vi "Get Wfm Logs.vi"(8 "error in (no error)":errorcluster, 11 "Waveform Receive in":refnum<class "Waveform Receive.lvclass">) -> (0 "error out":errorcluster, 2 "Associated Logs":T1[](array[typedef]), 3 "Waveform Receive out":refnum<class "Waveform Receive.lvclass">)   [LabVIEW 2015, in "Waveform Receive.lvclass"]
uses:
  Waveform Receive.lvclass
  Associated Log.ctl
  Waveform Receive.lvclass/Waveform Receive.ctl
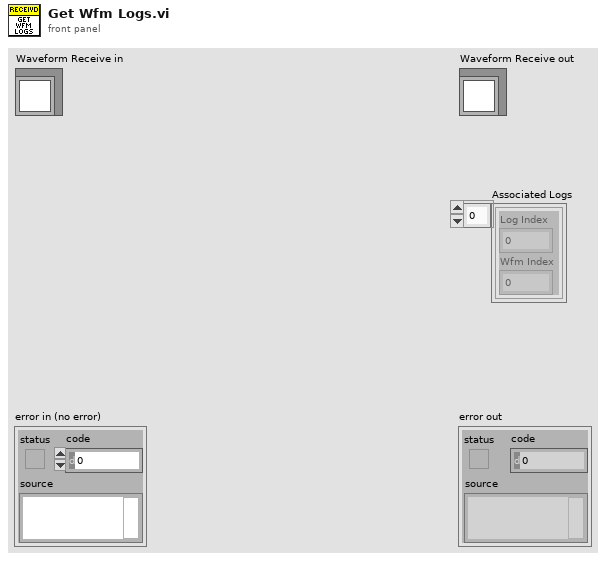
[diagram p1: front panel]
types:
  T1 = typedef "Waveform Receive.lvclass/Associated Log.ctl" = cluster{"Log Index":i32, "Wfm Index":i32}
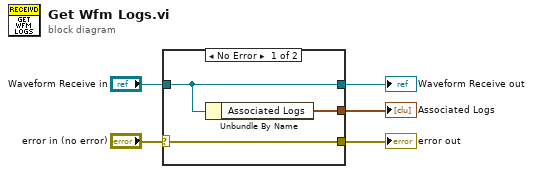
[diagram p0: block diagram]
diagram:
  n1 = case shown="No Error" "error in (no error)" {
    selector: "error in (no error)" -> [w8 w10]
    tunnel: [w8 w10] -> w4
    tunnel: [w7 w9] -> w2
    tunnel: "Waveform Receive in" -> [w7 w9]
    tunnel: [w6 _] -> w1
    frame No Error {
      n2 = Unbundle By Name(w7) -> ("Associated Logs"=w6:T1[])
    }
    frame Error {
    }
  }
  "error out" <- w4
  "Waveform Receive out" <- w2
  "Associated Logs" <- w1
